vi "Scale Matrix.vi"(2 "Scale":cluster{"X":dbl, "Y":dbl}={"X"=1.0, "Y"=1.0}, 3 "Matrix Type (2x2)":T1=[[1.0, 0.0], [0.0, 1.0]]) -> (1 "Matrix Out":T1)   [LabVIEW 2023, in "Font Glyph Drawer Interface.lvlib"]
uses:
  Font Glyph Drawer Interface.lvlib
  <vilib>/Analysis/Matrix/Datatypes/RealMatrix.ctl
  <vilib>/Analysis/Matrix/NI_Matrix.lvlib
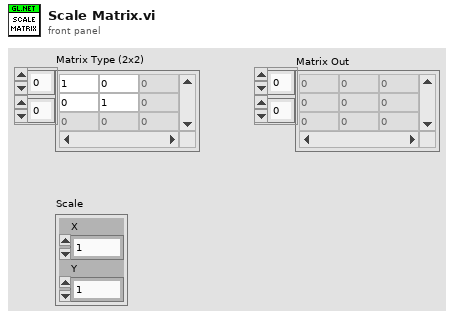
[diagram p1: front panel]
types:
  T1 = typedef "NI_Matrix.lvlib/RealMatrix.ctl" = dbl[][]
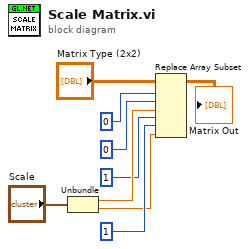
[diagram p0: block diagram]
diagram:
  n1 = Unbundle("Scale") -> ("X"=w5:dbl, "Y"=w2:dbl)
  n2 = Replace Array Subset(array="Matrix Type (2x2)", new element #1=w5, index (row) #1=0 ("index (row)"), index (col) #1=0 ("disabled index (col)"), new element #2=w2, index (row) #2=1 ("index (row)"), index (col) #2=1 ("disabled index (col)")) -> (→"Matrix Out":T1)
